vi "Copy Image to Memory Address.vi"   [LabVIEW 2020, in "image.lvlib"]
doc: "Copy the image source into the Memory Destination.\n\n<b>Ensure the Destination Parameters are correct to avoid memory corruption.</b>"
uses:
  image.lvlib
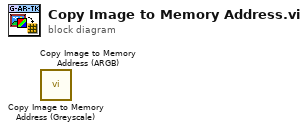
[diagram p0: block diagram]
diagram:
  n1 = call "Copy Image to Memory Address (Greyscale).vi"() -> ()  [unwired: 10 in, 2 out]
  n2 = call "Copy Image to Memory Address (ARGB).vi"() -> ()  [unwired: 10 in, 2 out]
